vi "GPS_SubVI.vi"(0 "read buffer":string) -> (1 "Number of satellites in use":dbl, 2 "Longitude":string, 3 "Latitude [deg]":string)   [LabVIEW 2015]
panel:
  out "Longitude [deg]":string
  out "Time":string
  in  "Time zone":i32
  out "Mode":string
  out "Date [ddmmyy]":string
  out "Course over ground [degrees]":string
  out "Speed over ground (knots)":string
  out "E/W":string
  out "N/S":string
  out "Latitude":string
  out "Status":string
  out "UTC Time":string
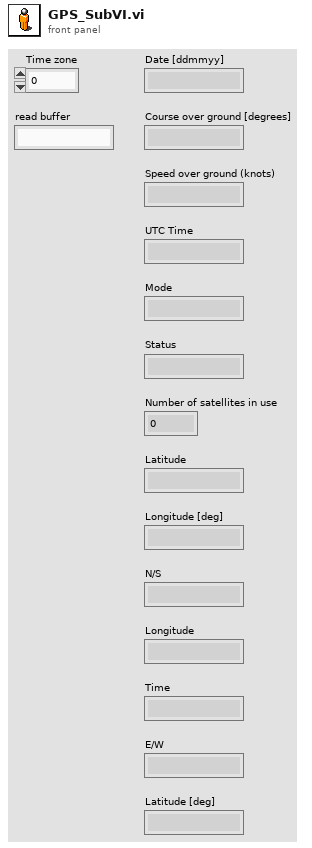
[diagram p1: front panel]
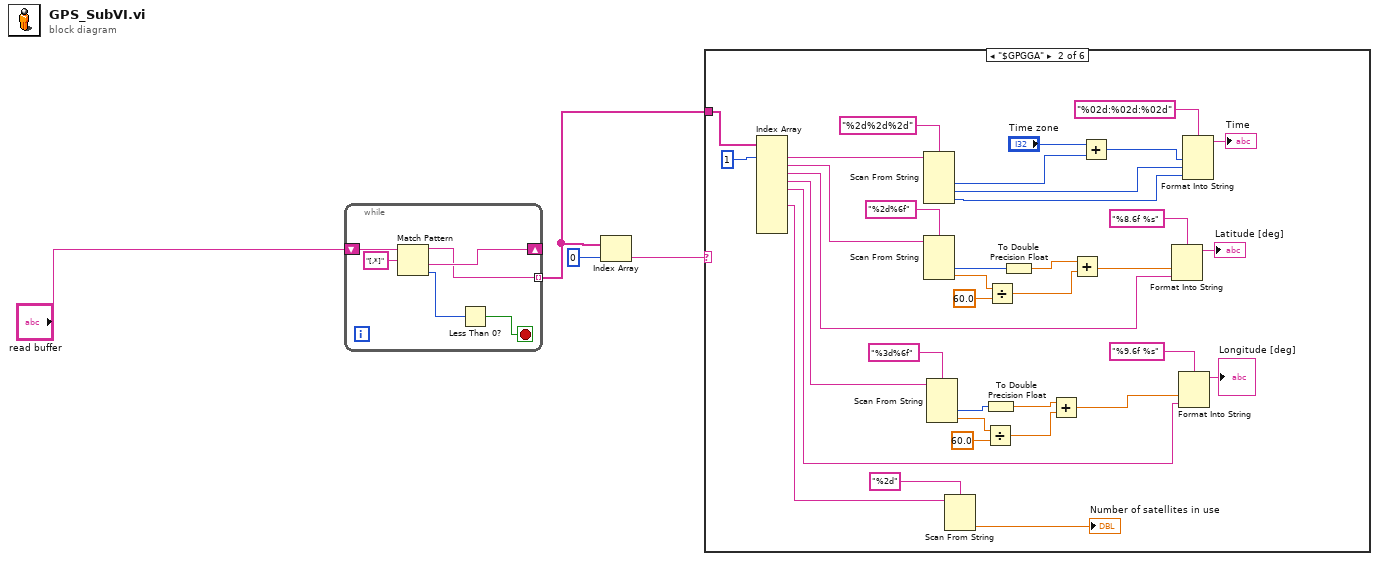
[diagram p0: block diagram]
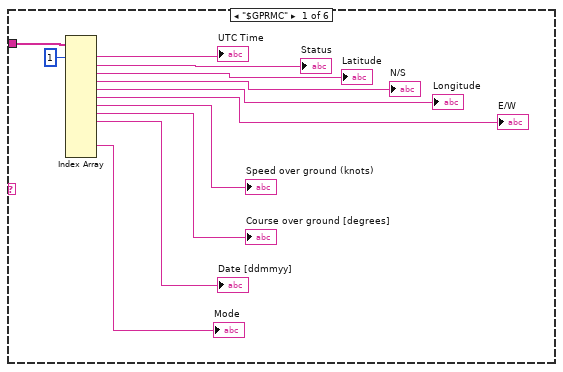
[diagram p2: hidden frame]
diagram:
  n1 = while {
    shift-right: [w6] -> _
    shift-left: "read buffer" -> [w10]
    tunnel: [w5] -> w4 mode=indexing
    stop <- w8 stop-if-true
    n2 = Match Pattern(string=w10, regular expression="[,*]") -> (before substring=w5:string, after substring=w6:string, offset past match=w7:i32)  [unwired: 1 in, 1 out]
    n3 = Less Than 0?(x=w7) -> (x < 0?=w8:bool)
  }
  n4 = Index Array(array=w4, index=0) -> (element=w3:string)
  n5 = case shown="\"$GPGGA\"" w3 {
    tunnel: w4 -> [w21 w58 _ _ _ _]
    frame "$GPRMC" {
      n6 = Index Array(array=w21, index #1=1 ("index")) -> (element #1=→"UTC Time":string, element #2=→"Status":string, element #3=→"Latitude":string, element #4=→"N/S":string, element #5=→"Longitude":string, element #6=→"E/W":string, element #7=→"Speed over ground (knots)":string, element #8=→"Course over ground [degrees]":string, element #9=→"Date [ddmmyy]":string, element #12=→"Mode":string)  [unwired: 12 in, 3 out]
    }
    frame "$GPGGA" {
      n7 = Index Array(array=w58, index #1=1 ("index")) -> (element #1=w56:string, element #2=w46:string, element #3=w38:string, element #4=w35:string, element #5=w29:string, element #7=w25:string)  [unwired: 9 in, 4 out]
      n8 = Scan From String(format string="%2d%2d%2d", input string=w56) -> (output 1=w54:i32, output 2=w51:i32, output 3=w48:i32)  [unwired: 5 in, 3 out]
      n9 = Scan From String(format string="%2d%6f", input string=w46) -> (output 1=w45:i32, output 2=w43:dbl)  [unwired: 4 in, 3 out]
      n10 = Scan From String(format string="%3d%6f", input string=w35) -> (output 1=w34:i32, output 2=w31:dbl)  [unwired: 4 in, 3 out]
      n11 = Scan From String(format string="%2d", input string=w25) -> (output 1=→"Number of satellites in use":dbl)  [unwired: 3 in, 3 out]
      n12 = Divide(x=w31, y=60.0) -> (x/y=w30:dbl)
      n13 = To Double Precision Float(number=w34) -> (double precision float=w33:dbl)
      n14 = Divide(x=w43, y=60.0) -> (x/y=w42:dbl)
      n15 = To Double Precision Float(number=w45) -> (double precision float=w41:dbl)
      n16 = Add(x=w33, y=w30) -> (x+y=w28:dbl)
      n17 = Add(x=w41, y=w42) -> (x+y=w39:dbl)
      n18 = Add(x="Time zone", y=w54) -> (x+y=w52:i32)
      n19 = Format Into String(format string="%8.6f %s", w39, w38) -> (resulting string=→"Latitude [deg]":string)  [unwired: 2 in, 1 out]
      n20 = Format Into String(format string="%9.6f %s", w28, w29) -> (resulting string=→"Longitude [deg]":string)  [unwired: 2 in, 1 out]
      n21 = Format Into String(format string="%02d:%02d:%02d", w52, w51, w48) -> (resulting string=→"Time":string)  [unwired: 2 in, 1 out]
    }
    frame "GPGSA" {
    }
    frame "$GPGSV" {
    }
    frame "$GPVTG" {
    }
    frame Default {
    }
  }
